vi "PluginsLoaderCommander_SendStop.vi"(8 "error in (no error)":errorcluster, 11 "PluginsLoaderCommander in":refnum<class "PluginsLoaderCommander.lvclass">) -> (0 "error out":errorcluster, 3 "PluginsLoaderCommander out":refnum<class "PluginsLoaderCommander.lvclass">)   [LabVIEW 2014, in "PluginsThread.lvlib" / "PluginsLoaderCommander.lvclass"]
uses:
  PluginsLoaderCommander.lvclass
  PluginsLoaderCommander_CommandData.ctl
  PluginsLoaderCommander_Command.ctl
  PluginsLoaderCommander.lvclass/PluginsLoaderCommander.ctl
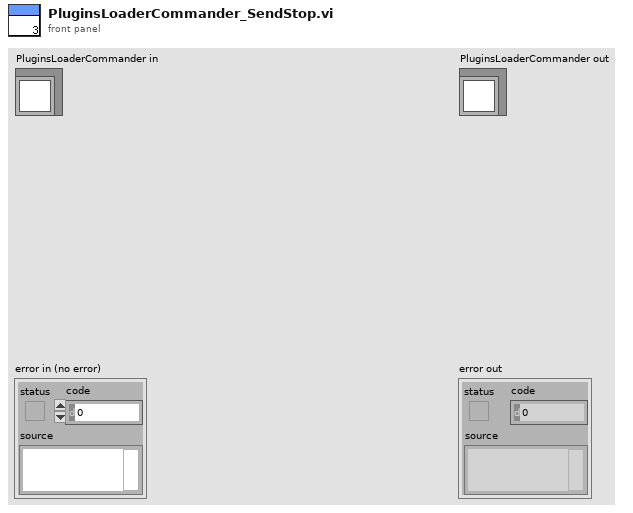
[diagram p1: front panel]
types:
  T1 = typedef "PluginsThread.lvlib/PluginsLoaderCommander.lvclass/PluginsLoaderCommander_Command.ctl" = enum16{"Stop", "Timeout"}
  T2 = typedef "PluginsThread.lvlib/PluginsLoaderCommander.lvclass/PluginsLoaderCommander_CommandData.ctl" = cluster{"Command":T1, "Data":variant}
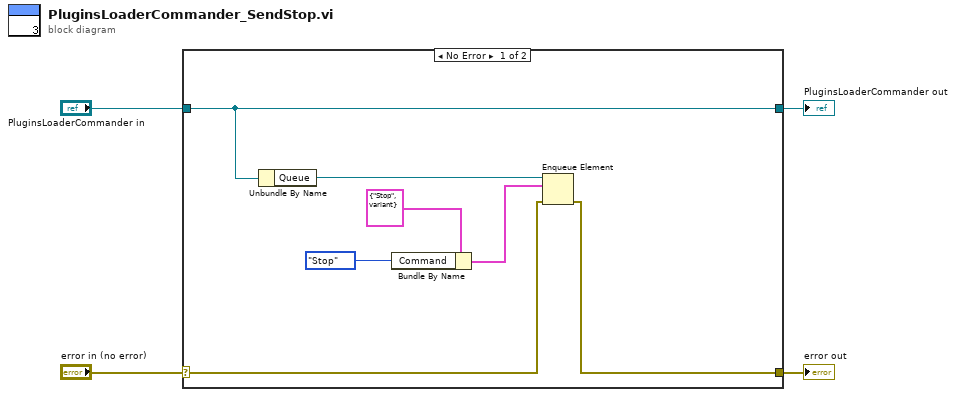
[diagram p0: block diagram]
diagram:
  n1 = case shown="No Error" "error in (no error)" {
    selector: "error in (no error)" -> [w7 w13]
    tunnel: [w6 w13] -> w3
    tunnel: [w11 w12] -> w1
    tunnel: "PluginsLoaderCommander in" -> [w11 w12]
    frame No Error {
      n2 = Unbundle By Name(w11) -> ("Queue"=w10:refnum<queue>)
      n3 = Bundle By Name(cluster=T2 {"Command"=enum."Stop", "Data"=variant} ("element"), "Command"=PluginsLoaderCommander_Command."Stop") -> (w8:T2)
      n4 = Enqueue Element(queue=w10, element=w8, error in (no error)=w7) -> (error out=w6:errorcluster)  [unwired: 1 in, 2 out]
    }
    frame Error {
    }
  }
  "error out" <- w3
  "PluginsLoaderCommander out" <- w1
